vi "DLTS - timing calculation (SubVI).vi"   [LabVIEW 2019]
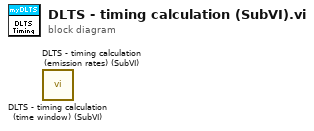
[diagram p0: block diagram]
diagram:
  n1 = call "DLTS - timing calculation (time window) (SubVI).vi"() -> ()  [unwired: 12 in, 4 out]
  n2 = call "DLTS - timing calculation (emission rates) (SubVI).vi"() -> ()  [unwired: 12 in, 4 out]
